vi "What is Arround Me.vi"(3 "What?Midbrain":cluster{"T":dbl, "Range":dbl, "Bearing":dbl}[](array[cluster])) -> (1 "What?Midbrain 2":cluster{"T":dbl, "Range":dbl, "Bearing":dbl}[](array[cluster]))   [LabVIEW 2010]
doc: "This SubVI takes clean Whatsense data from the Midbrain and layers perception onto it to be passed to the THINK processes in the Forebrain\n\nT=time\nRange\nBearing"
uses:
  5.0-Global.vi
panel:
  out "What?Forebrain":cluster{"T":dbl, "Range":dbl, "Bearing":dbl}[](array[cluster])
  out "What?Midbrain 3":cluster{"T":dbl, "Range":dbl, "Bearing":dbl}[](array[cluster])
  out "AutoModeLIDAR":picture
  # "This SubVI adds \nperception onto the\nWhere data comming\nfrom the Midbrain"
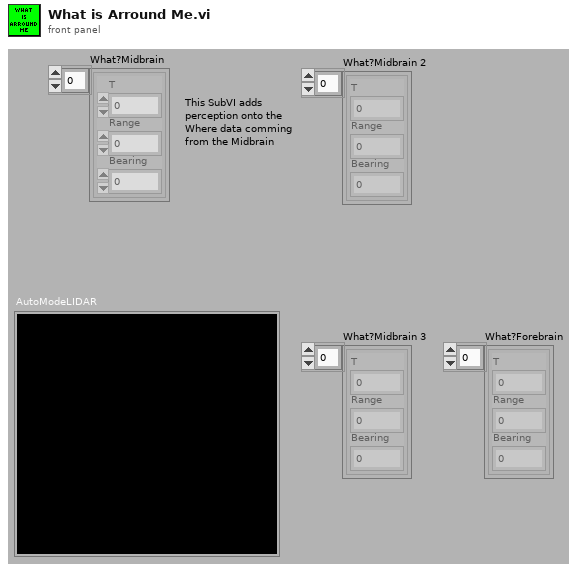
[diagram p1: front panel]
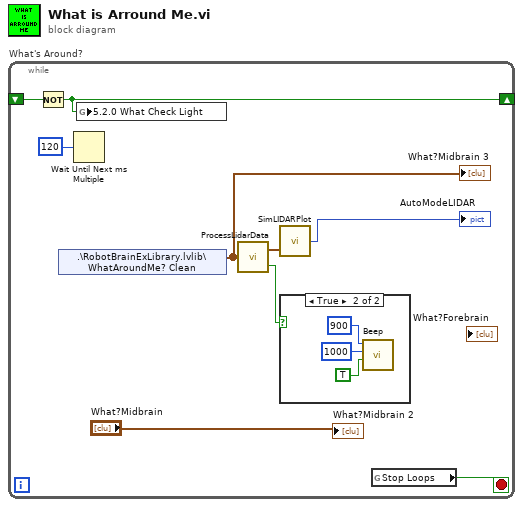
[diagram p0: block diagram]
diagram:
  n1 = while "What's Around?" {
    shift-right: [w3] -> _
    shift-left: _ -> [w8]
    stop <- w4 stop-if-true
    n2 = Not(x=w8) -> (.not. x?=w3:bool)
    n3 = shared-variable ".\\RobotBrainExLibrary.lvlib\\WhatAroundMe? Clean"() -> (w7:cluster{"T":dbl, "Range":dbl, "Bearing":dbl}[])  [unwired: 1 in, 1 out]
    "What?Midbrain 3" <- w7
    n4 = Wait Until Next ms Multiple(millisecond multiple=u32 120 ("milliseconds to wait")) -> ()  [unwired: 1 out]
    n5 = global write "5.0-Global.vi" "5.2.0 What Check Light"(w3) -> ()
    n6 = call "ProcessLidarData.vi"("WhatAroundMe?MM"=w7) -> ("Collision"=w5:bool, "data array [mag, phase (deg)]"=w2:cluster{"magnitude":dbl, "phase":dbl}[])
    n7 = call "SimLIDARPlot.vi"("data array [mag, phase (deg)]"=w2) -> ("SONAR"=→"AutoModeLIDAR":picture)  [unwired: 1 in]
    n8 = case shown="True" w5 {
      frame False {
        # "No \nBeep"
      }
      frame True {
        n9 = call <vilib>:"Beep.vi"("use system alert? (T)"=TRUE, "duration (msec)"=u32 1000, "frequency (Hz)"=u32 900) -> ()  [unwired: 9 in]
      }
    }
    n10 = global read "5.0-Global.vi" "Stop Loops"() -> (w4:bool)
    "What?Midbrain 2" <- "What?Midbrain"
  }
